vi "Fetch Data & Offsets.vi"(4 "Include Command":bool=TRUE, 5 "Include Reading":bool, 6 "Source":T1, 7 "Force Tag":string) -> (0 "Cartesian Offsets":dbl[][](array[numeric]), 1 "Cartesian Data":dbl[][](array[numeric]), 2 "Actuator Offsets":dbl[][](array[numeric]), 3 "Actuator Data":dbl[][](array[numeric]))   [LabVIEW 2009]
uses:
  Transactions/Dataset Source.ctl
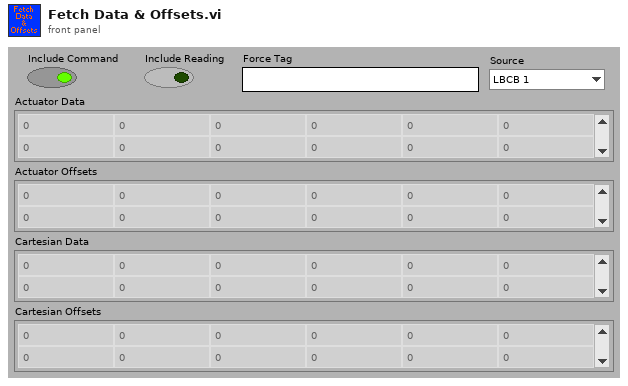
[diagram p1: front panel]
types:
  T1 = typedef "Dataset Source.ctl" = enum16{"LBCB 1", "LBCB 2", "Combined", "External Sensors"}
  T2 = typedef "Dataset Transaction Id.ctl" = cluster{"Dataset Source":T1, "Dataset Type":T3, "Hold":T4, "Volts":T4, "Tag":string}
  T3 = typedef "Dataset Type.ctl" = enum16{"LVDT", "Load Cell", "Actuator Command", "Servo Error", "Displacement Command", "Displacement", "Force"}
  T4 = typedef "Yes No Button.ctl" = bool
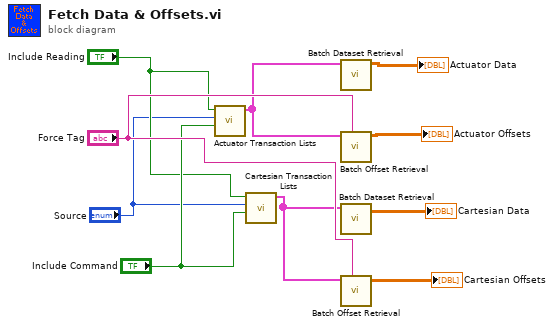
[diagram p0: block diagram]
diagram:
  n1 = call "Actuator Transaction Lists.vi"("Include Command"="Include Command", "Source"="Source", "Include Reading"="Include Reading") -> ("Actuator Data"=w4:T2[])  [unwired: 2 in, 2 out]
  n2 = call "Cartesian Transaction Lists.vi"("Include Command"="Include Command", "Source"="Source", "Include Reading"="Include Reading") -> ("Transactions"=w8:T2[])  [unwired: 3 in, 1 out]
  n3 = call "Batch Dataset Retrieval.vi"("Transactions"=w4) -> ("Data"=→"Actuator Data":dbl[][])  [unwired: 9 in, 1 out]
  n4 = call "Batch Offset Retrieval.vi"("Tag"="Force Tag", "Transactions"=w4) -> ("Data"=→"Actuator Offsets":dbl[][])  [unwired: 8 in, 1 out]
  n5 = call "Batch Dataset Retrieval.vi"("Transactions"=w8) -> ("Data"=→"Cartesian Data":dbl[][])  [unwired: 9 in, 1 out]
  n6 = call "Batch Offset Retrieval.vi"("Tag"="Force Tag", "Transactions"=w8) -> ("Data"=→"Cartesian Offsets":dbl[][])  [unwired: 8 in, 1 out]
